vi "HasTransitionFailed.vi"() -> (3 "HasTransitionFailed?":bool)   [LabVIEW 2013]
doc: "This VI should check whether the boat has failed the transition it is in, and it should only be called if the boat is currently in a transition state.\n\nAt the moment the thought is that only a tack can fail, jibes and turning without crossing the wind should never be ruled as failed. This is because in a jibe or turn there is always force on the boat to let it keep trying to turn, and in a tack if the boat gets stuck in irons there isn't any useful force on the boat. At that point keeping on trying to turn won't get anywhere, and a 'failed' flag should be raised.\n\nEric Schneider, Feb, 2014"
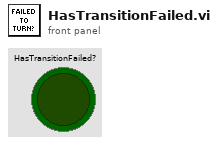
[diagram p1: front panel]
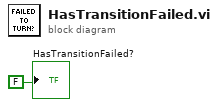
[diagram p0: block diagram]
diagram:
  "HasTransitionFailed?" <- FALSE ("HasTransitionFailed?")
